vi "AddUIBusy.vi"(11 "State in":string) -> (3 "State out":string)   [LabVIEW 2016, in "LabVIEWCodeCoverage.lvlib"]
uses:
  LabVIEWCodeCoverage.lvlib
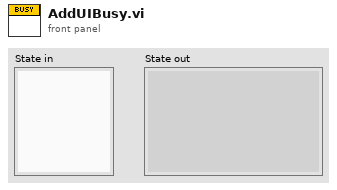
[diagram p1: front panel]
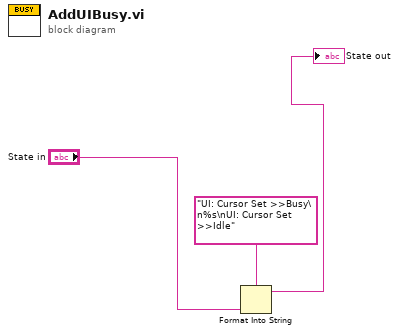
[diagram p0: block diagram]
diagram:
  n1 = Format Into String(format string="UI: Cursor Set >>Busy\n%s\nUI: Cursor Set >>Idle", "State in") -> (resulting string=→"State out":string)  [unwired: 2 in, 1 out]
